vi "Read ScanCode.vi"(8 "error in (no error)":errorcluster, 11 "ControlKeyDownMsg in":refnum<class "ControlKeyDownMsg.lvclass">) -> (0 "error out":errorcluster, 2 "ScanCode":i16, 3 "ControlKeyDownMsg out":refnum<class "ControlKeyDownMsg.lvclass">)   [LabVIEW 2017, in "ActorEvents.lvlib" / "ControlKeyDownMsg.lvclass"]
uses:
  ControlKeyDownMsg.lvclass
  ControlKeyDownMsg.lvclass/ControlKeyDownMsg.ctl
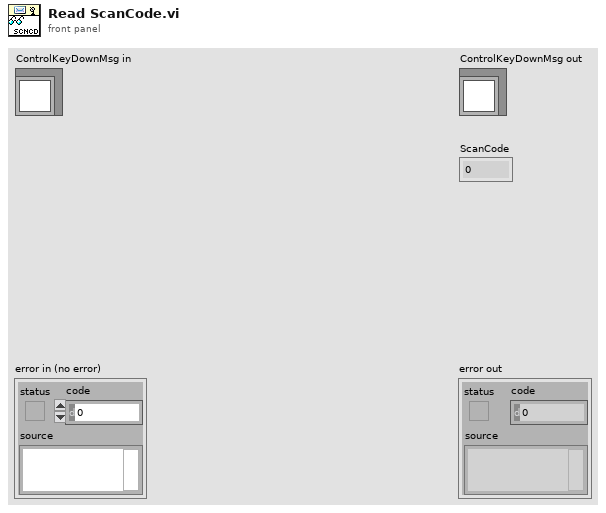
[diagram p1: front panel]
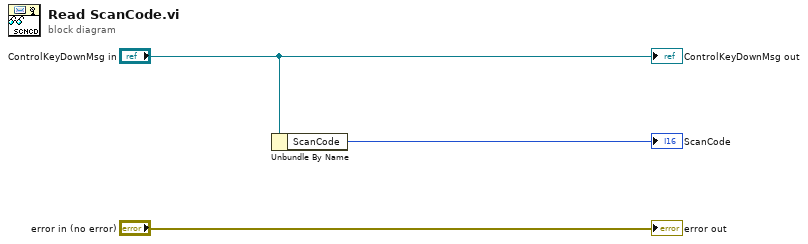
[diagram p0: block diagram]
diagram:
  n1 = Unbundle By Name("ControlKeyDownMsg in") -> ("ScanCode"=→"ScanCode":i16)
  "error out" <- "error in (no error)"
  "ControlKeyDownMsg out" <- "ControlKeyDownMsg in"
